vi "host test SPI IP .vi"() -> ()   [LabVIEW 2014]
uses:
  <userlib>/_NI SPI IP/FPGA/Controllers/Public/Spi Master Inputs.ctl
  <userlib>/_NI SPI IP/FPGA/Controllers/Public/Transfer Settings.ctl
  <userlib>/_NI SPI IP/FPGA/Controllers/NI SPI IP FPGA.lvlib
panel:
  out "CS":cluster{i16, i16, i16}(graph)
  out "Waveform Chart":i16(graph)
  in  "spi transfer settings":T1={"Divide Value"=39, "Transfer Length (bits)"=24, "CS Asserted Polarity"=FALSE, "Clock Polarity (CPOL)"=FALSE, "Clock Phase (CPHA)"=FALSE, "Lengthen MISO Setup"=FALSE, "Direction Change Bit"=0, "MOSI Starts as Output"=FALSE, "Tristatable MOSI"=FALSE} {"Direction Change Bit" max=64 step=1; "Transfer Length (bits)" min=1 max=64 step=1}
  in  "data to write":u64 format="%.0x"
  in  "spi input":T2
  in  "Boolean":bool
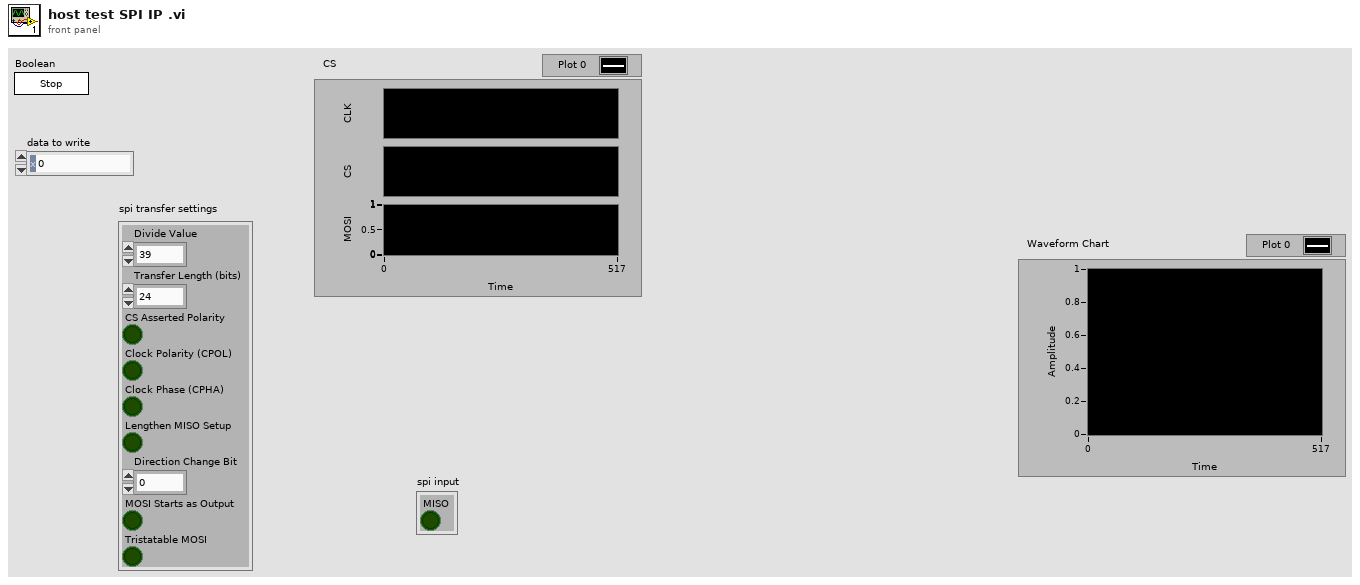
[diagram p1: front panel]
types:
  T1 = typedef "NI SPI IP FPGA.lvlib/Transfer Settings.ctl" = cluster{"Divide Value":u8, "Transfer Length (bits)":u8, "CS Asserted Polarity":bool, "Clock Polarity (CPOL)":bool, "Clock Phase (CPHA)":bool, "Lengthen MISO Setup":bool, "Direction Change Bit":u8, "MOSI Starts as Output":bool, "Tristatable MOSI":bool}
  T2 = typedef "NI SPI IP FPGA.lvlib/Spi Master Inputs.ctl" = cluster{"MISO":bool}
  T3 = typedef "NI SPI IP FPGA.lvlib/Spi Master Outputs.ctl" = cluster{"Chip Select":bool, "Clock":bool, "MOSI":bool, "MOSI OE":bool}
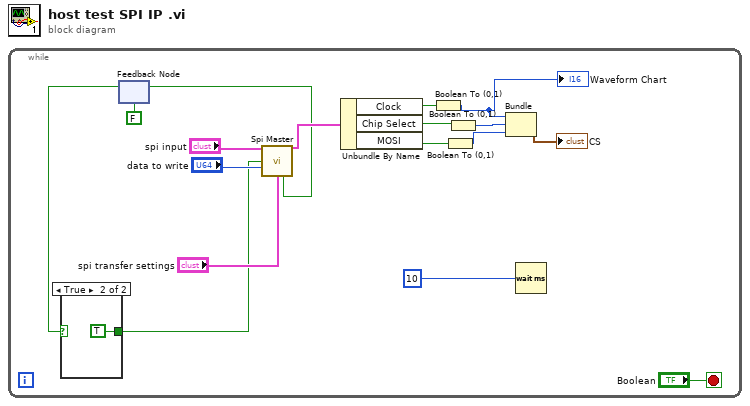
[diagram p0: block diagram]
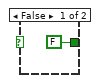
[diagram p2: hidden frame]
diagram:
  n1 = while {
    stop <- "Boolean" stop-if-true
    n2 = feedback #1(FALSE ("ready for input")) -> (w2:bool)
    n3 = case shown="True" w2 {
      tunnel: [FALSE TRUE] -> w4
      frame False {
      }
      frame True {
      }
    }
    n4 = call <userlib>:"Spi Master.vi"("spi input"="spi input", "start strobe"=w4, "data to write"="data to write", "spi transfer settings"="spi transfer settings") -> ("spi output"=w14:T3, "ready for input"=w3:bool)  [unwired: 8 in, 2 out]
    n5 = feedback-in #1(w3) -> ()
    n6 = Unbundle By Name(w14) -> ("Clock"=w10:bool, "Chip Select"=w12:bool, "MOSI"=w5:bool)
    n7 = Boolean To (0,1)(Boolean=w10) -> (0, 1=w9:i16)
    "Waveform Chart" <- w9
    n8 = Boolean To (0,1)(Boolean=w5) -> (0, 1=w6:i16)
    n9 = Boolean To (0,1)(Boolean=w12) -> (0, 1=w8:i16)
    n10 = Bundle(w9, w8, w6) -> (→"CS":cluster{i16, i16, i16})  [unwired: 1 in]
    n11 = Wait (ms)(milliseconds to wait=u32 10) -> ()  [unwired: 1 out]
  }
